vi "NATS Client Unit Test.vi"() -> (0 "error out":errorcluster)   [LabVIEW 2024]
uses:
  <vilib>/addons/_JKI Toolkits/Caraya/classes/Test/Test.lvclass
  NATS Client/NATS Client.lvclass
  <vilib>/addons/_JKI Toolkits/Caraya/classes/Assert/Assert.lvclass
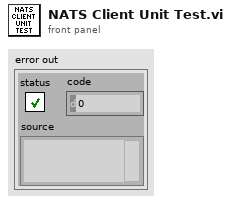
[diagram p1: front panel]
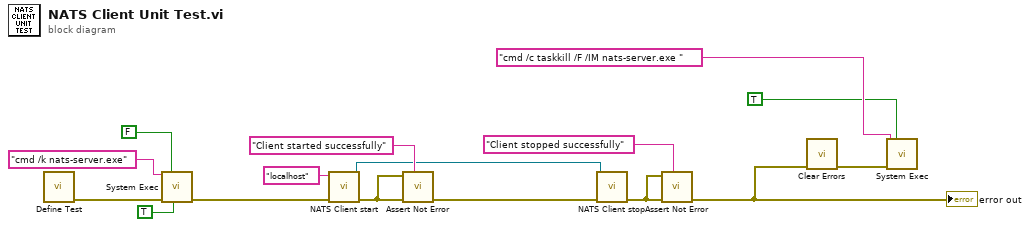
[diagram p0: block diagram]
diagram:
  n1 = call <vilib>:"Define Test.vi"() -> ("error out"=w11:errorcluster)  [unwired: 10 in, 1 out]
  n2 = call <vilib>:"System Exec.vi"("run minimized? (F)"=TRUE, "wait until completion? (T)"=FALSE, "error in (no error)"=w11, "command line"="cmd /k nats-server.exe") -> ("error out"=w10:errorcluster)  [unwired: 4 in, 3 out]
  n3 = call "NATS Client start.vi"("error in"=w10, "address"="localhost") -> ("error out"=w15:errorcluster, "NATS Client out"=w4:refnum<class "NATS Client.lvclass">)  [unwired: 8 in]
  n4 = call <vilib>:"Assert Not Error.vi"("Label"="Client started successfully", "error in (no error)"=w15, "Not Error?"=w15) -> ("error out"=w5:errorcluster)  [unwired: 7 in, 1 out]
  n5 = call "NATS Client stop.vi"("error in"=w5, "NATS Client"=w4) -> ("error out"=w13:errorcluster)  [unwired: 9 in]
  n6 = call <vilib>:"Assert Not Error.vi"("Label"="Client stopped successfully", "error in (no error)"=w13, "Not Error?"=w13) -> ("error out"=w7:errorcluster)  [unwired: 7 in, 1 out]
  "error out" <- w7
  n7 = call <vilib>:"Clear Errors.vi"("error in (no error)"=w7) -> ("error out"=w6:errorcluster)  [unwired: 5 in, 1 out]
  n8 = call <vilib>:"System Exec.vi"("wait until completion? (T)"=TRUE, "error in (no error)"=w6, "command line"="cmd /c taskkill /F /IM nats-server.exe ") -> ()  [unwired: 5 in, 4 out]
